vi "获取IP.vi"() -> (0 "IP地址":string)   [LabVIEW 2016]
panel:
  out "字符串":string
  out "MAC地址":string
  out "standard output":string caption="标准输出"
  out "输出字符串":string
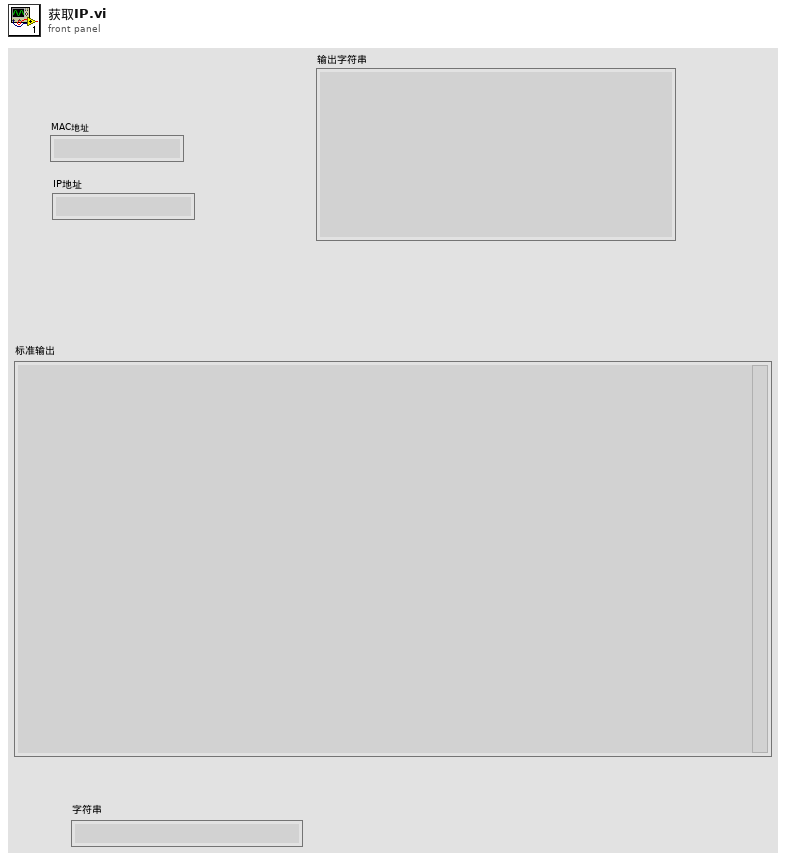
[diagram p1: front panel]
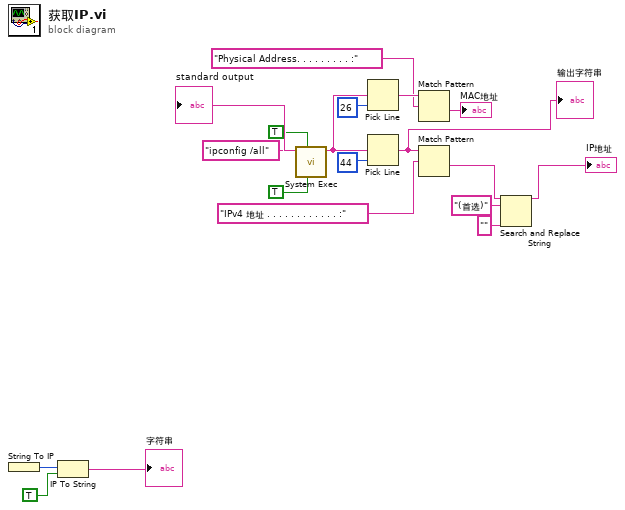
[diagram p0: block diagram]
diagram:
  n1 = String To IP() -> (0:w2:u32)  [unwired: 1 in]
  n2 = IP To String(1:TRUE ("句点符号？(F)"), 2:w2) -> (0:→"字符串":string)
  n3 = call <vilib>:"System Exec.vi"("run minimized? (F)"=TRUE, "wait until completion? (T)"=TRUE, "command line"="ipconfig /all") -> ("standard output"=w16:string)  [unwired: 3 in, 5 out]
  "standard output" <- w16
  n4 = Pick Line(multi-line string=w16, line index=26) -> (output string=w14:string)  [unwired: 1 out]
  n5 = Pick Line(multi-line string=w16, line index=44) -> (output string=w18:string)  [unwired: 1 out]
  "输出字符串" <- w18
  n6 = Match Pattern(string=w14, regular expression="Physical Address. . . . . . . . . :") -> (after substring=→"MAC地址":string)  [unwired: 4 out]
  n7 = Match Pattern(string=w18, regular expression="IPv4 地址 . . . . . . . . . . . . :") -> (after substring=w7:string)  [unwired: 4 out]
  n8 = Search and Replace String(input string=w7, search string="(首选)" ("搜索字符串"), replace string="" ("替换字符串(\"\")")) -> (result string=→"IP地址":string)  [unwired: 5 in, 3 out]
